vi "Joystick Multipliers.vi"(6 "z axis":dbl, 8 "error in (no error)":errorcluster, 9 "y axis":dbl, 10 "x axis":dbl, 11 "throttle":dbl) -> (0 "error out":errorcluster, 1 "y out":dbl, 2 "x out":dbl, 4 "z out":dbl)   [LabVIEW 2014]
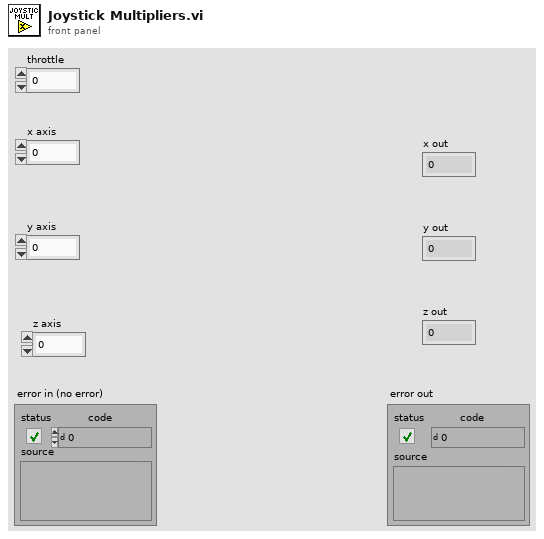
[diagram p1: front panel]
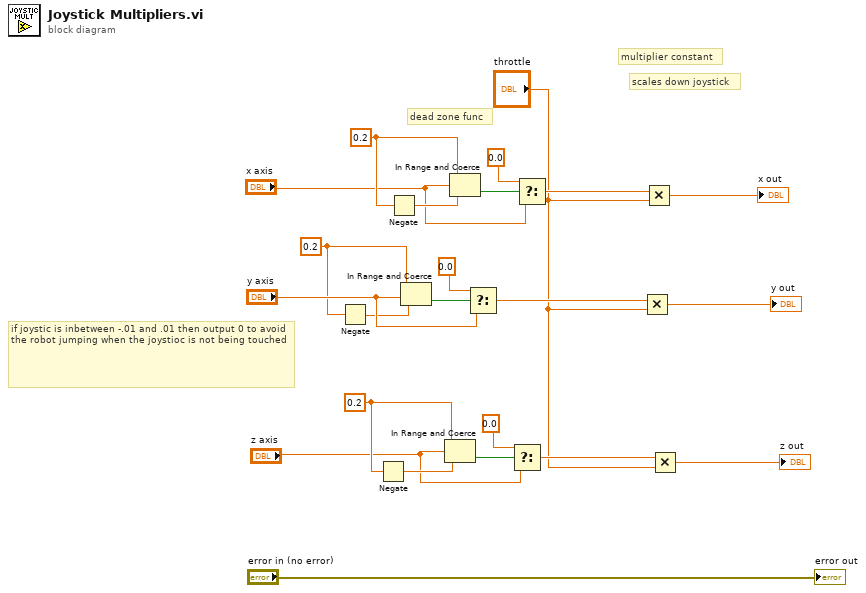
[diagram p0: block diagram]
diagram:
  w7 = 0.2 ("lower limit")
  w13 = 0.2 ("lower limit")
  w2 = 0.2 ("lower limit")
  # "scales down joystick"
  # "if joystic is inbetween -.01 and .01 then output 0 to avoid the robot jumping when the joystioc is not being touched"
  # "dead zone func"
  # "multiplier constant"
  n1 = Negate(x=w2) -> (-x=w15:dbl)
  n2 = Negate(x=w7) -> (-x=w8:dbl)
  n3 = Negate(x=w13) -> (-x=w14:dbl)
  n4 = In Range and Coerce(upper limit=w2, x="y axis", lower limit=w15) -> (In Range?=w19:bool)  [unwired: 1 out]
  n5 = In Range and Coerce(upper limit=w7, x="z axis", lower limit=w8) -> (In Range?=w5:bool)  [unwired: 1 out]
  n6 = In Range and Coerce(upper limit=w13, x="x axis", lower limit=w14) -> (In Range?=w11:bool)  [unwired: 1 out]
  n7 = Select(t=0.0 ("f"), s=w19, f="y axis") -> (s? t:f=w16:dbl)
  n8 = Select(t=0.0 ("f"), s=w5, f="z axis") -> (s? t:f=w4:dbl)
  n9 = Select(t=0.0 ("f"), s=w11, f="x axis") -> (s? t:f=w9:dbl)
  n10 = Multiply(x=w16, y="throttle") -> (x*y=→"y out":dbl)
  n11 = Multiply(x=w9, y="throttle") -> (x*y=→"x out":dbl)
  n12 = Multiply(x=w4, y="throttle") -> (x*y=→"z out":dbl)
  "error out" <- "error in (no error)"
